vi "Resize.vi"   [LabVIEW 2020, in "image.lvlib"]
doc: "Resize the image source into the destination."
uses:
  image.lvlib
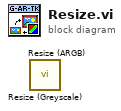
[diagram p0: block diagram]
diagram:
  n1 = call "Resize (Greyscale).vi"() -> ()  [unwired: 10 in, 2 out]
  n2 = call "Resize (ARGB).vi"() -> ()  [unwired: 10 in, 2 out]
